vi "AO.vi"(10 "模拟输出通道设置":T1={"数据输出通道设置"={"maximum value"=5.0, "minimum value"=-5.0, "input terminal configuration"=-1, "physical channels"=""}, "采样设置"={"rate"=1000.0, "sample mode"=10178, "samples per channel"=1000}, "ConvLateErrorsToWarnings"=FALSE} {"采样设置"."sample mode" items=["Finite Samples"=10178, "Continuous Samples"=10123, "Hardware Timed Single Point"=12522]; "采样设置"."rate" format="%0.2f"; "数据输出通道设置"."input terminal configuration" items=["Default"=-1, "RSE"=10083, "NRSE"=10078, "Differential"=10106, "Pseudodifferential"=12529]; "数据输出通道设置"."minimum value" format="%0.2f"; "数据输出通道设置"."maximum value" format="%0.2f"}) -> (0 "error out":errorcluster, 3 "task out":refnum<k21>)   [LabVIEW 2018]
uses:
  <vilib>/DAQmx/create/channels.llb/DAQmx Create Channel (AO-Voltage-Basic).vi
  <vilib>/DAQmx/configure/timing.llb/DAQmx Timing (Sample Clock).vi
  <resource>/objmgr/daqmx.rc
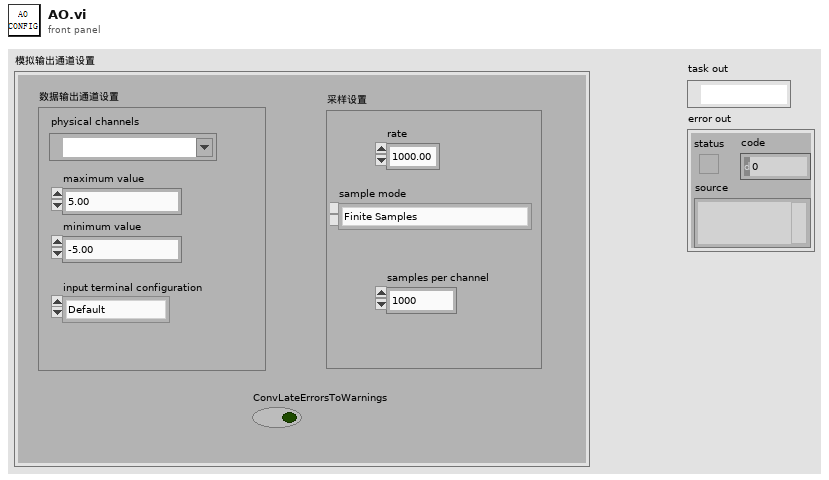
[diagram p1: front panel]
types:
  T1 = cluster{"数据输出通道设置":cluster{"maximum value":dbl, "minimum value":dbl, "input terminal configuration":i32, "physical channels":tag}, "采样设置":cluster{"rate":dbl, "sample mode":i32, "samples per channel":i32}, "ConvLateErrorsToWarnings":bool}
  T2 = cluster{"rate":dbl, "sample mode":i32, "samples per channel":i32}
  T3 = cluster{"maximum value":dbl, "minimum value":dbl, "input terminal configuration":i32, "physical channels":tag}
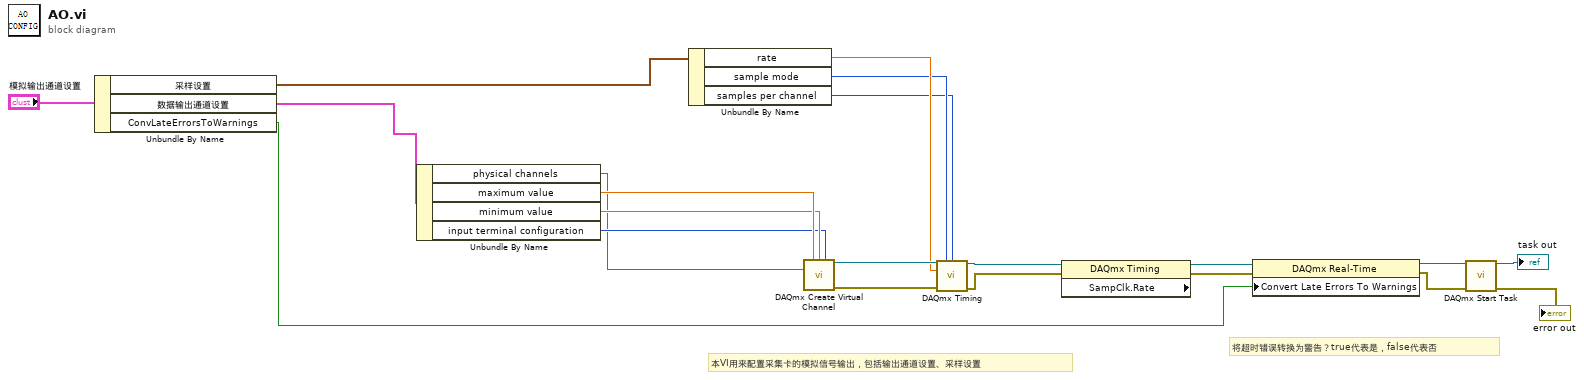
[diagram p0: block diagram]
diagram:
  # "将超时错误转换为警告？true代表是，false代表否"
  # "本VI用来配置采集卡的模拟信号输出，包括输出通道设置、采样设置"
  n1 = Unbundle By Name("模拟输出通道设置") -> ("采样设置"=w3:T2, "数据输出通道设置"=w2:T3, "ConvLateErrorsToWarnings"=w1:bool)
  n2 = Unbundle By Name(w2) -> ("physical channels"=w5:tag, "maximum value"=w11:dbl, "minimum value"=w10:dbl, "input terminal configuration"=w9:i32)
  n3 = Unbundle By Name(w3) -> ("rate"=w8:dbl, "sample mode"=w7:i32, "samples per channel"=w6:i32)
  n4 = call-poly <vilib>:"DAQmx Create Virtual Channel.vi"("maximum value"=w11, "minimum value"=w10, "output terminal configuration"=w9, "physical channels"=w5) -> ("task out"=w19:refnum<k21>, "error out"=w18:errorcluster)  [unwired: 10 in]
  n5 = call-poly <vilib>:"DAQmx Timing.vi"("task/channels in"=w19, "sample mode"=w7, "samples per channel"=w6, "rate"=w8, "error in"=w18) -> ("task out"=w17:refnum<k21>, "error out"=w16:errorcluster)  [unwired: 9 in]
  n6 = property class="DAQmx Timing" props=["SampClk.Rate"](reference=w17, error in=w16) -> (reference out=w21:refnum<k21>, error out=w20:errorcluster)  [unwired: 1 out]
  n7 = property class="DAQmx Real-Time"(reference=w21, error in=w20, "Convert Late Errors To Warnings"=w1) -> (reference out=w15:refnum<k21>, error out=w14:errorcluster)
  n8 = call <vilib>:"DAQmx Start Task.vi"("task/channels in"=w15, "error in"=w14) -> ("task out"=→"task out":refnum<k21>, "error out"=→"error out":errorcluster)  [unwired: 12 in]
